vi "Show UI.vi"(0 "object in":refnum<class "IManager.lvclass">, 2 "UI Type":T1, 5 "Error In":errorcluster) -> (14 "object out":refnum<class "IManager.lvclass">, 19 "Error Out":errorcluster)   [LabVIEW 2024, in "IManager.lvclass"]
doc: "Shows selected UI type"
uses:
  IManager.lvclass
  UIType.ctl
panel:
  # "Connector Pane"
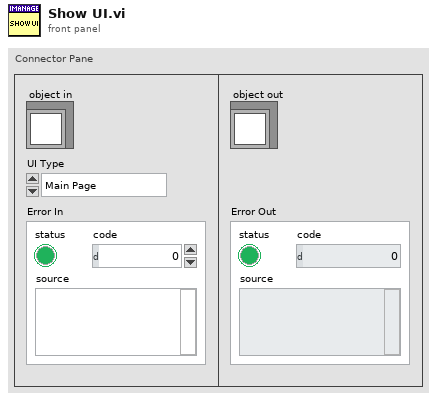
[diagram p1: front panel]
types:
  T1 = typedef "UIType.ctl" = enum16{"Main Page", "Settings Page", "Debugging Page"}
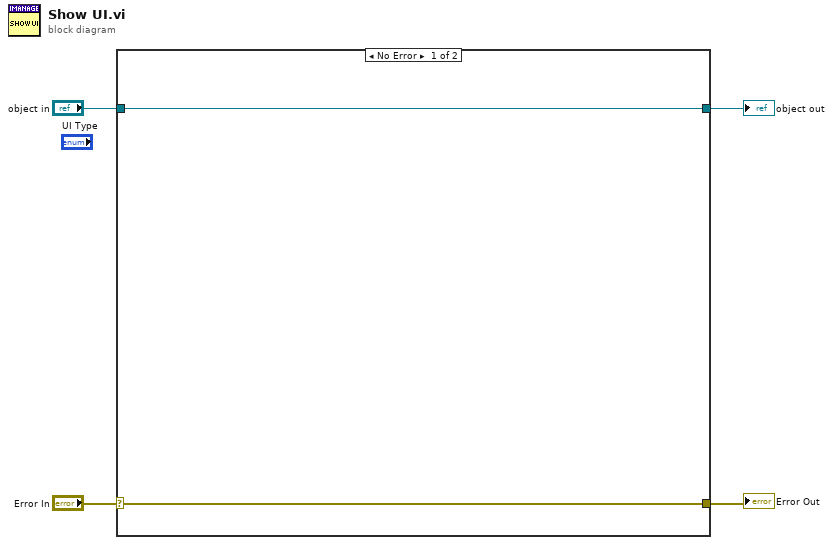
[diagram p0: block diagram]
diagram:
  n1 = case shown="No Error" "Error In" {
    selector: "Error In" -> [w5 w8]
    tunnel: [w5 w8] -> w3
    tunnel: [w6 w7] -> w1
    tunnel: "object in" -> [w6 w7]
    frame No Error {
    }
    frame Error {
    }
  }
  "Error Out" <- w3
  "object out" <- w1
